vi "setParameters.vi"(10 "Parameters":T1, 11 "TestAirCommand in":refnum<class "TestAirCommand.lvclass">) -> (3 "TestAirCommand out":refnum<class "TestAirCommand.lvclass">)   [LabVIEW 2016, in "TestAirCommand.lvclass"]
uses:
  TestAirCommand.lvclass
  DataTypes/Topics/CommandTestAir.ctl
  DataTypes/Topics/Parts/CommandId.ctl
  TestAirCommand.lvclass/TestAirCommand.ctl
  DataTypes/Topics/M1M3SupportTopics.lvlib
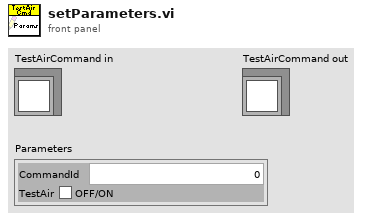
[diagram p1: front panel]
types:
  T1 = typedef "M1M3SupportTopics.lvlib/CommandTestAir.ctl" = cluster{"CommandId":T2, "TestAir":bool}
  T2 = typedef "M1M3SupportTopics.lvlib/CommandId.ctl" = i32
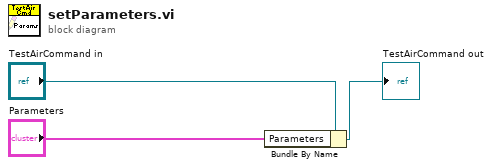
[diagram p0: block diagram]
diagram:
  n1 = Bundle By Name(cluster="TestAirCommand in", "Parameters"="Parameters") -> (→"TestAirCommand out":refnum<class "TestAirCommand.lvclass">)
